vi "GainMultiply1.vi"(0 "Gain Exponent":i8, 5 "Gain":fxp<+/-,18,1> format="%.18g", 9 "Input":fxp<+/-,18,1> format="%.18g", 12 "Unique 8b identifier":u8) -> (3 "Timed out":bool, 8 "Output":fxp<+/-,18,1> format="%.18g", 14 "Unexponentiated Output":fxp<+/-,18,1> format="%.18g")   [LabVIEW 2010]
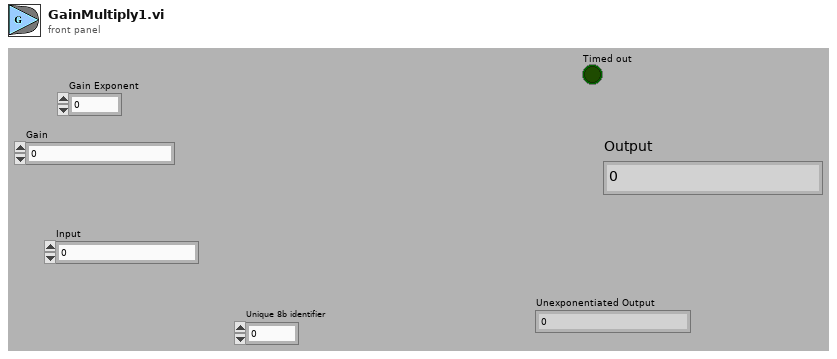
[diagram p1: front panel]
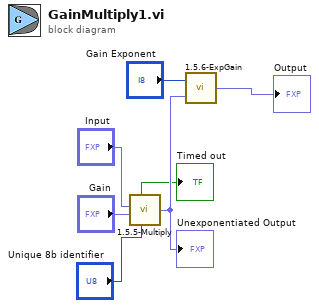
[diagram p0: block diagram]
diagram:
  n1 = call "1.5.5-Multiply.vi"("Input A"="Input", "Input B"="Gain", "Unique 8b identifier"="Unique 8b identifier") -> ("Timed out"=→"Timed out":bool, "Output"=w3:fxp<+/-,18,1>)  [unwired: 4 in]
  "Unexponentiated Output" <- w3
  n2 = call "1.5.6-ExpGain.vi"("18b (s-fxp-1) in"=w3, "N"="Gain Exponent") -> ("18b (s-fxp-1) out"=→"Output":fxp<+/-,18,1>)
